vi "Gyroscope.vi"(0 "State Control":enum16{"Open", "Run", "End"}(ring)) -> (1 "Angle":dbl(knob) scale=0.0..360.0, 2 "Initial Position?":bool)   [LabVIEW 2013]
doc: "Gyro Example\n\nThis VI shows the user how to open a channel to a Gyro, get an angle from a gyro, and reinitialize the gyro."
uses:
  <vilib>/Rock Robotics/SystemInterfaces/AI/FPGA_AIGyroChannel.ctl
panel:
  in  "Gain (VoltsPerDegree/Second)":dbl=0.006675 format="%#_13g"
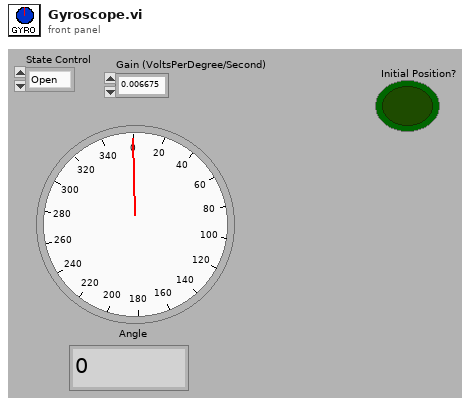
[diagram p1: front panel]
types:
  T1 = typedef "FPGA_AIGyroChannel.ctl" = enum8{"AI 1", "AI 2", "Invalid"}
  T2 = typedef "WPI_GyroDevRef.ctl" = cluster{"DevStatus":errorcluster, "Analog Module":T3, "Analog Channel":T4, "Offset":dbl, "Gain (VoltsPerDegree/Second)":dbl}
  T3 = typedef "FPGA_TypedefAnalogModule.ctl" = enum16{"Analog Module 1", "Analog Module 2"}
  T4 = typedef "FPGA_AIChannel.ctl" = enum8{"AI 1", "AI 2", "AI 3", "AI 4", "AI 5", "AI 6", "AI 7", "AI 8", "Invalid"}
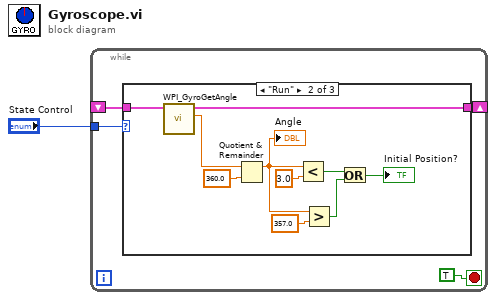
[diagram p0: block diagram]
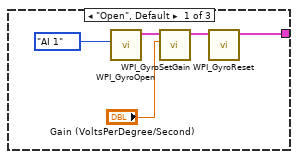
[diagram p2: hidden frame]
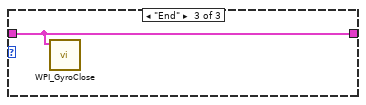
[diagram p3: hidden frame]
diagram:
  n1 = while {
    tunnel: "State Control" -> [w5]
    shift-right: [w3] -> _
    shift-left: _ -> [w2]
    stop <- TRUE stop-if-true
    n2 = case shown="\"Run\"" w5 {
      tunnel: [w6 w17 w21] -> w3
      tunnel: w2 -> [_ w20 w21]
      frame "Open", Default {
        n3 = call <vilib>:"WPI_GyroOpen.vi"("Analog Channel"=FPGA_AIGyroChannel."AI 1" ("Channel")) -> ("GyroDevRef"=w10:T2)  [unwired: 5 in, 5 out]
        n4 = call <vilib>:"WPI_GyroSetGain.vi"("Gain (VoltsPerDegree/Second)"="Gain (VoltsPerDegree/Second)", "GyroDevRef"=w10) -> ("GyroDevRef"=w7:T2)  [unwired: 1 in, 8 out]
        n5 = call <vilib>:"WPI_GyroReset.vi"("GyroDevRef"=w7) -> ("GyroDevRef"=w6:T2)  [unwired: 10 out]
      }
      frame "Run" {
        n6 = call <vilib>:"WPI_GyroGetAngle.vi"("GyroDevRef"=w20) -> ("Angle"=w18:dbl, "GyroDevRef"=w17:T2)  [unwired: 1 in, 8 out]
        n7 = Quotient & Remainder(x=w18, y=360.0) -> (x-y*floor(x/y)=w15:dbl)  [unwired: 1 out]
        "Angle" <- w15
        n8 = Less?(x=w15, y=3.0) -> (x < y?=w13:bool)
        n9 = Greater?(x=w15, y=357.0) -> (0:w12:bool)
        n10 = Or(x=w13, y=w12) -> (x .or. y?=→"Initial Position?":bool)
      }
      frame "End" {
        n11 = call <vilib>:"WPI_GyroClose.vi"("GyroDevRef"=w21) -> ()  [unwired: 1 in, 10 out]
      }
    }
  }
